vi "Read Stock Trader.vi"(8 "error in (no error)":errorcluster, 11 "Order in":refnum<class "Order.lvclass">) -> (0 "error out":errorcluster, 2 "Stock Trader":refnum<class "Stock Trader.lvclass">, 3 "Order out":refnum<class "Order.lvclass">)   [LabVIEW 2019, in "Order.lvclass"]
doc: "Access the stock trader (receiver) object that is used to execute this order (command)"
uses:
  Order.lvclass
  Stock Trader/Stock Trader.lvclass
  Order.lvclass/Order.ctl
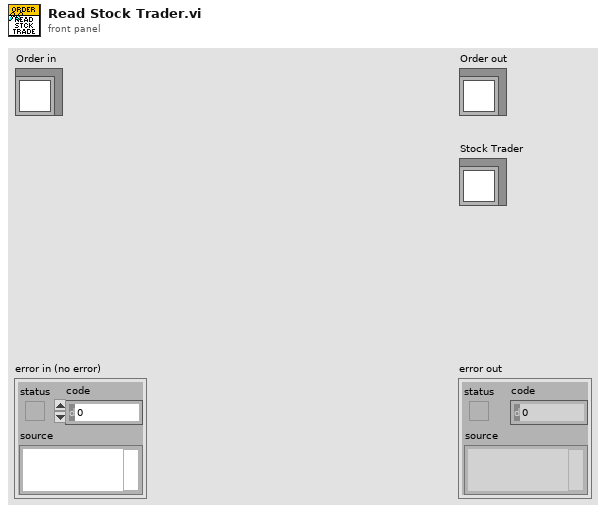
[diagram p1: front panel]
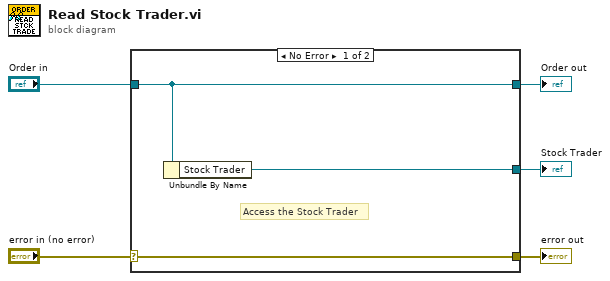
[diagram p0: block diagram]
diagram:
  n1 = case shown="No Error" "error in (no error)" {
    selector: "error in (no error)" -> [w8 w9]
    tunnel: [w8 w9] -> w4
    tunnel: [w7 w10] -> w2
    tunnel: "Order in" -> [w7 w10]
    tunnel: [w6 _] -> w1
    frame No Error {
      # "Access the Stock Trader"
      n2 = Unbundle By Name(w7) -> ("Stock Trader"=w6:refnum<class "Stock Trader.lvclass">)
    }
    frame Error {
    }
  }
  "error out" <- w4
  "Order out" <- w2
  "Stock Trader" <- w1
